vi "LVClass_WavefrontCorrectorSet Write WavefrontCorrectorSet.vi"(8 "error in (no error)":errorcluster, 10 "WavefrontCorrectorSet":i32, 11 "WavefrontCorrectorSet in":refnum<class "WavefrontCorrectorSet.lvclass">) -> (0 "error out":errorcluster, 3 "WavefrontCorrectorSet out":refnum<class "WavefrontCorrectorSet.lvclass">)   [LabVIEW 2020, in "WavefrontCorrectorSet.lvclass"]
uses:
  WavefrontCorrectorSet.lvclass
  WavefrontCorrectorSet.lvclass/WavefrontCorrectorSet.ctl
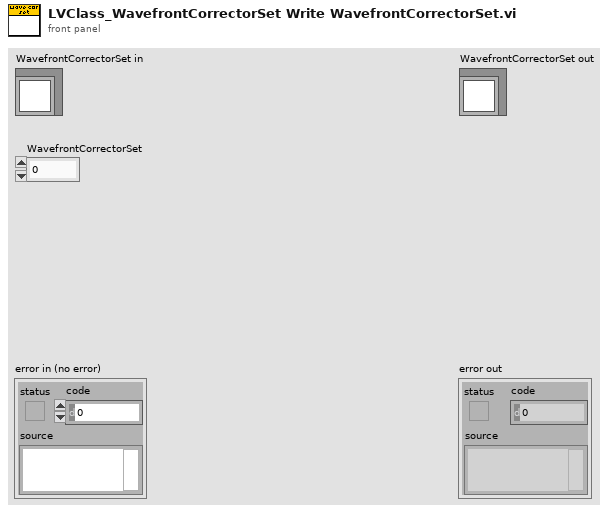
[diagram p1: front panel]
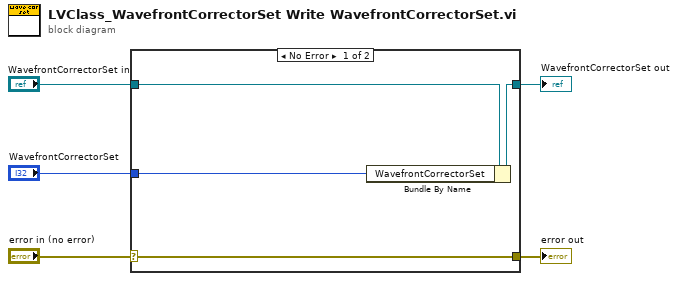
[diagram p0: block diagram]
diagram:
  n1 = case shown="No Error" "error in (no error)" {
    selector: "error in (no error)" -> [w9 w10]
    tunnel: [w9 w10] -> w4
    tunnel: [w7 w11] -> w2
    tunnel: "WavefrontCorrectorSet in" -> [w8 w11]
    tunnel: "WavefrontCorrectorSet" -> [w6 _]
    frame No Error {
      n2 = Bundle By Name(cluster=w8, "WavefrontCorrectorSet"=w6) -> (w7:refnum<class "WavefrontCorrectorSet.lvclass">)
    }
    frame Error {
    }
  }
  "error out" <- w4
  "WavefrontCorrectorSet out" <- w2
